vi "FPGA_lock-in_analysis-light.vi"() -> ()   [LabVIEW 2010]
uses:
  <vilib>/eio/EIONode/EIONode.xnode
  <vilib>/LabVIEW Targets/FPGA/cRIO/shared/nicrio_ModuleControls/nicrio_cRIO-9205_VoltageRange.ctl
  <vilib>/eio/EIOMethodNode/EIOMethodNode.xnode
  <vilib>/rvi/DataTransferAndStorage/Container/XNode/niFpgaContainer.xnode
  <vilib>/rvi/FIFO/Fifo_Resource/nirvififoEmulationSetSize.vi
  <vilib>/rvi/DataTransferAndStorage/Container/Common/niFpgaContainerGetUniqueNameForEmu.vi
  <vilib>/rvi/DataTransferAndStorage/Container/Common/niFpgaTransferTypeControl.ctl
  <vilib>/rvi/DataTransferAndStorage/Container/Common/niFpgaContainerMethod.ctl
  <vilib>/rvi/interface/RandomDataEmulation/nirviRandomDataFPGAFIFO.vi
  <vilib>/rvi/interface/RandomDataEmulation/niFpgaRandomDataHandleErrors.vi
panel:
  in  "data-sent-to-host":enum8{"LI", "average"}(ring)
  in  "dt/tau":fxp<+,25,0>
  in  "Voltage Range":T1
  in  "lock-in input channel":u8 max=31 step=1
  out "XXX lock-in IN":fxp<+/-,26,5> format="%.23g"
  # "dt is the time between two points ( @ 250 kSample/s )"
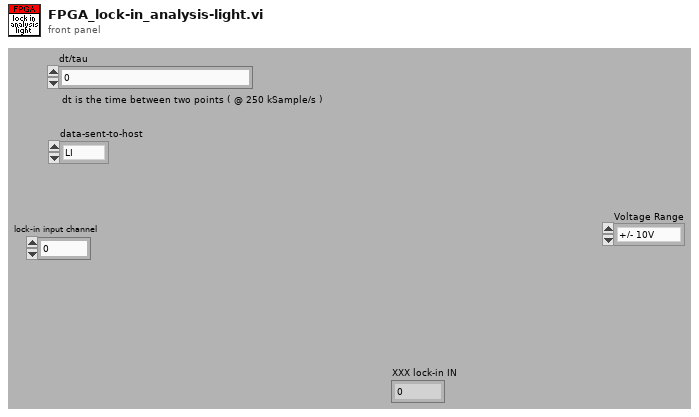
[diagram p1: front panel]
types:
  T1 = typedef "nicrio_cRIO-9205_VoltageRange.ctl" = enum8{"+/- 10V", "+/- 5V", "+/- 1V", "+/- 200mV"}
  T2 = typedef "niFpgaContainerMethod.ctl" = enum16{"<none>", "write", "read", "clear", "getNumberOfElementsToWrite", "getNumberOfElementsToRead", "enable", "disable", "flushAndDisable", "getStreamState", "readA", "readB", "dramWrite", "dramWriteWithByteEnables", "dramRequestData", "dramRetrieveData"}
  T3 = typedef "niFpgaTransferTypeControl.ctl" = enum16{"Target-Scoped", "Host to Target - DMA", "Target to Host - DMA", "Peer to Peer Reader", "Peer to Peer Writer", "Bidirectional"}
  T4 = cluster{"Boolean array[0]":bool, "Boolean array[1]":bool}
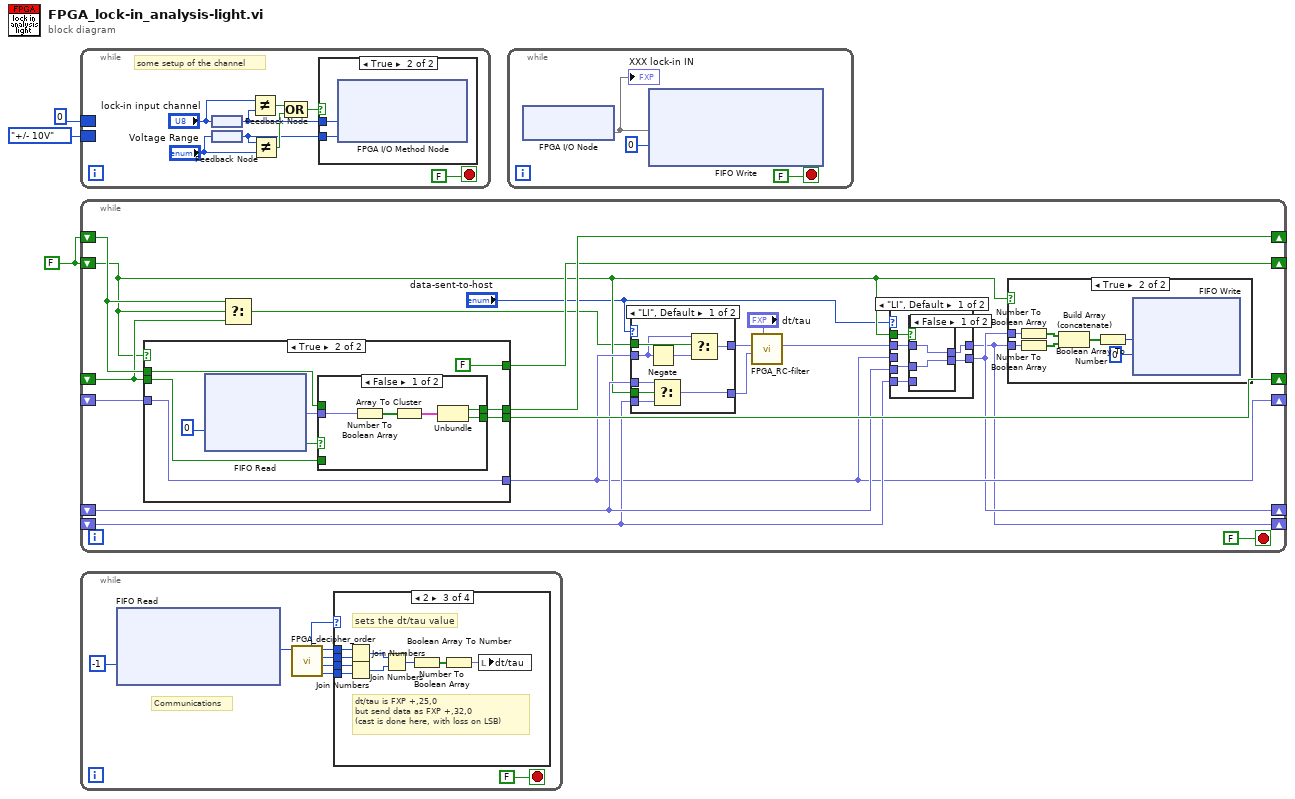
[diagram p0: block diagram]
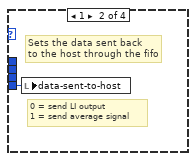
[diagram p3: hidden frame]
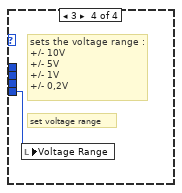
[diagram p4: hidden frame]
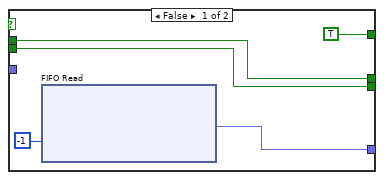
[diagram p10: hidden frame]
diagram:
  w1 = FALSE
  n1 = while {
    border: u8 0 ("AI Channel") -> [_]
    border: nicrio_cRIO-9205_VoltageRange."+/- 10V" ("Voltage Range") -> [_]
    stop <- FALSE stop-if-true
    # "some setup of the channel"
    n2 = feedback-in #1("lock-in input channel") -> ()
    n3 = feedback #1() -> (w10:u8)
    n4 = feedback-in #2("Voltage Range") -> ()
    n5 = feedback #2() -> (w5:T1)
    n6 = Not Equal?(x="lock-in input channel", y=w10) -> (x != y?=w8:bool)
    n7 = Not Equal?(x=w5, y="Voltage Range") -> (x != y?=w9:bool)
    n8 = Compound Arithmetic op=OR(w8, w9) -> (w7:bool)
    n9 = case shown="True" w7 {
      tunnel: w5 -> [_ w13]
      tunnel: w10 -> [_ w12]
      frame False {
      }
      frame True {
        n10 = xnode "FPGA I/O Method Node"("AI Channel"=w12, "Voltage Range"=w13) -> ()  [unwired: 1 in, 1 out]
      }
    }
  }
  n11 = while {
    shift-right: [w31] -> _
    shift-left: w1 -> [w26]
    shift-right: [w30] -> _
    shift-left: _ -> [w25]
    shift-right: [w18] -> _
    shift-left: _ -> [w22]
    shift-right: [w14] -> _
    shift-left: _ -> [w21]
    shift-right: [w27] -> _
    shift-left: w1 -> [w19]
    shift-right: [w20] -> _
    shift-left: _ -> [w16]
    stop <- FALSE stop-if-true
    n12 = case shown="True" w19 {
      tunnel: [w93 w151] -> w31
      tunnel: [w92 w150] -> w30
      tunnel: w25 -> [w92 w149]
      tunnel: w26 -> [w93 w148]
      tunnel: [w90 w146] -> w20
      tunnel: [TRUE FALSE] -> w27
      tunnel: w16 -> [_ w146]
      frame False {
        n13 = xnode ("FIFO Read")("Timeout"=-1) -> ("Element"=w90:fxp<+/-,26,5>)  [unwired: 1 in, 2 out]
      }
      frame True {
        n14 = xnode ("FIFO Read")("Timeout"=0) -> ("Element"=w152:fxp<+,2,2>, "Timed Out?"=w153:bool)  [unwired: 1 in, 1 out]
        n15 = case shown="False" w153 {
          tunnel: w152 -> [w210 _]
          tunnel: [w207 w212] -> w151
          tunnel: [w206 w211] -> w150
          tunnel: w148 -> [_ w212]
          tunnel: w149 -> [_ w211]
          frame False {
            n16 = Number To Boolean Array(number=w210) -> (Boolean array=w209:bool[])
            n17 = Array To Cluster(array=w209) -> (cluster=w208:T4)
            n18 = Unbundle(w208) -> ("Boolean array[0]"=w207:bool, "Boolean array[1]"=w206:bool)
          }
          frame True {
          }
        }
      }
    }
    n19 = Select(t=w26, s=w19, f=w25) -> (s? t:f=w15:bool)
    n20 = case shown="\"LI\", Default" "data-sent-to-host" {
      tunnel: [w80 w88] -> w29
      tunnel: w20 -> [w82 w88]
      tunnel: [w87 w89] -> w24
      tunnel: w19 -> [w86 _]
      tunnel: w22 -> [w85 _]
      tunnel: w21 -> [w84 w89]
      tunnel: w15 -> [w83 _]
      frame "LI", Default {
        n21 = Negate(x=w82) -> (-x=w81:fxp<+/-,27,6>)
        n22 = Select(t=w85, s=w86, f=w84) -> (s? t:f=w87:fxp<+/-,32,5>)
        n23 = Select(t=w82, s=w83, f=w81) -> (s? t:f=w80:fxp<+/-,27,6>)
      }
      frame "average" {
      }
    }
    n24 = call "FPGA_RC-filter.vi"("deltaT/tau"="dt/tau", "X_n"=w24, "mesure"=w29) -> ("X_n+1"=w23:fxp<+/-,32,5>)  [unwired: 8 out]
    n25 = case shown="\"LI\", Default" "data-sent-to-host" {
      tunnel: w19 -> [w73 _]
      tunnel: w23 -> [w72 w79]
      tunnel: [w71 w78] -> w18
      tunnel: [w70 w79] -> w14
      tunnel: w22 -> [w69 _]
      tunnel: w21 -> [w68 _]
      tunnel: w20 -> [_ w78]
      frame "LI", Default {
        n26 = case shown="False" w73 {
          tunnel: w72 -> [w75 w77]
          tunnel: [w74 w77] -> w71
          tunnel: [w75 w76] -> w70
          tunnel: w69 -> [w74 _]
          tunnel: w68 -> [_ w76]
          frame False {
          }
          frame True {
          }
        }
      }
      frame "average" {
      }
    }
    n27 = case shown="True" w19 {
      tunnel: w18 -> [_ w37]
      tunnel: w14 -> [_ w36]
      frame False {
      }
      frame True {
        n28 = Number To Boolean Array(number=w37) -> (Boolean array=w35:bool[])
        n29 = Number To Boolean Array(number=w36) -> (Boolean array=w34:bool[])
        n30 = Build Array (concatenate)(w35, w34) -> (w33:bool[])
        n31 = Boolean Array To Number(Boolean array=w33) -> (number=w38:u64)
        n32 = xnode ("FIFO Write")("Element"=w38, "Timeout"=0) -> ()  [unwired: 1 in, 2 out]
      }
    }
  }
  n33 = while {
    stop <- FALSE stop-if-true
    # "Communications"
    n34 = xnode ("FIFO Read")("Timeout"=-1) -> ("Element"=w218:u64)  [unwired: 1 in, 2 out]
    n35 = call "FPGA_decipher_order.vi"("order in"=w218) -> ("data 1"=w216:u8, "data 2"=w215:u8, "data 3"=w214:u8, "data 4"=w213:u8, "order out"=w217:u8)  [unwired: 6 out]
    n36 = case shown="2" w217 {
      tunnel: w216 -> [_ w272 w278 w282]
      tunnel: w215 -> [_ _ w279 _]
      tunnel: w214 -> [_ _ w280 _]
      tunnel: w213 -> [_ _ w281 _]
      frame 0, Default {
      }
      frame 1 {
        # "0 = send LI output\n1 = send average signal"
        # "Sets the data sent back \nto the host through the fifo"
        n37 = local write "data-sent-to-host"(w272) -> ()
      }
      frame 2 {
        # "dt/tau is FXP +,25,0\nbut send data as FXP +,32,0\n(cast is done here, with loss on LSB)"
        # "sets the dt/tau value"
        n38 = Join Numbers(hi=w281, lo=w280) -> ((hi.lo)=w276:u16)
        n39 = Join Numbers(hi=w279, lo=w278) -> ((hi.lo)=w277:u16)
        n40 = Join Numbers(hi=w276, lo=w277) -> ((hi.lo)=w275:u32)
        n41 = Number To Boolean Array(number=w275) -> (Boolean array=w274:bool[])
        n42 = Boolean Array To Number(Boolean array=w274) -> (number=w273:fxp<+/-,32,0>)
        n43 = local write "dt/tau"(w273) -> ()
      }
      frame 3 {
        # "sets the voltage range :\n+/- 10V\n+/- 5V\n+/- 1V\n+/- 0,2V"
        # "set voltage range"
        n44 = local write "Voltage Range"(w282) -> ()
      }
    }
  }
  n45 = while {
    stop <- FALSE stop-if-true
    n46 = xnode "FPGA I/O Node"() -> ("ModA/AI0"=w283)  [unwired: 1 in, 1 out]
    "XXX lock-in IN" <- w283
    n47 = xnode ("FIFO Write")("Element"=w283, "Timeout"=0) -> ()  [unwired: 1 in, 2 out]
  }
